vi "SMO.Dictionary.GetValue.vi"(6 "timeout (10ms)":i32=10, 8 "error in (no error)":errorcluster, 10 "Key":string, 11 "SMO.Dictionary":refnum<class "SMO.Dictionary.lvclass">) -> (0 "error out":errorcluster, 1 "Value":variant, 2 "Key":string, 3 "SMO.Dictionary out":refnum<class "SMO.Dictionary.lvclass">, 4 "timed out?":bool)   [LabVIEW 2013, in "SMO.Dictionary.lvlib" / "SMO.Dictionary.lvclass"]
doc: "---------------------------------------------------------------\nJKI State Machine Objects™\nhttp://jki.net/state-machine-objects/\nCopyright (C) 2005-2015, JKI <info@jki.net>\nALL RIGHTS RESERVEDJKI State Machine Objects (SMO) 1.0.0.4\nJKI - JKI\nCopyright (c) 2015, JKI"
uses:
  SMO.Dictionary.lvclass
  Typedefs/PrivateEvents--SMO.Dictionary.Get.ctl
  Typedefs/PrivateEvents--SMO.Dictionary.KeyValue-Pair.ctl
  <vilib>/JKI/JKI SMO/SMO/SMO.lvclass
panel:
  # "For instructions on how to use the JKI State Machine Objects, examples and video tutorials, visit:\nhttp://jki.net/state-machine-objects/\n\nJKI State Machine Objects™\nhttp://jki.net/state-machine-objects/\nCopyright (C) 2005-2015, JKI <info@jki.net>\nALL RIGHTS RESERVED"
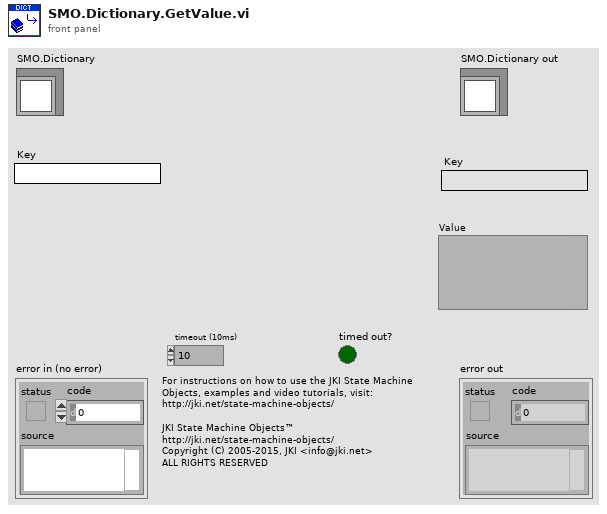
[diagram p1: front panel]
types:
  T1 = typedef "SMO.lvclass/SMOState --Enum.ctl" = enum16{"unknown", "Created", "Started", "Stopped"}
  T2 = typedef "SMO.Dictionary.lvlib/SMO.Dictionary.lvclass/PrivateEvents--SMO.Dictionary.KeyValue-Pair.ctl" = cluster{"Key":string, "Value":variant}
  T3 = typedef "SMO.Dictionary.lvlib/SMO.Dictionary.lvclass/PrivateEvents--SMO.Dictionary.Get.ctl" = cluster{"Key":string, "response":refnum<notifier>}
  T4 = typedef "SMO.Dictionary.lvlib/SMO.Dictionary.lvclass/PrivateEvents--Cluster.ctl" = cluster{"Update":refnum<user-event>, "Clear Dictionary":refnum<user-event>, "Delete":refnum<user-event>, "Get":refnum<user-event>, "GetMultiple":refnum<user-event>}
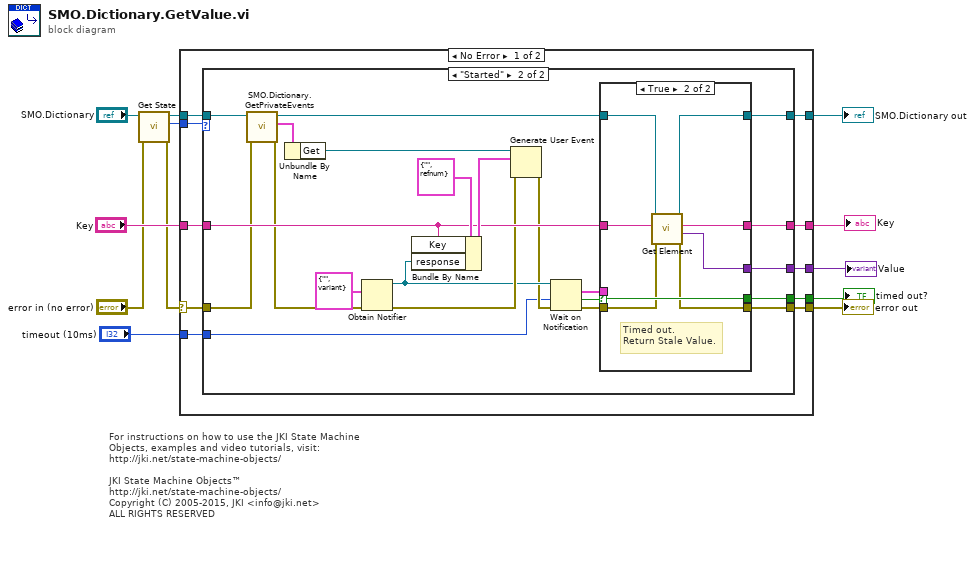
[diagram p0: block diagram]
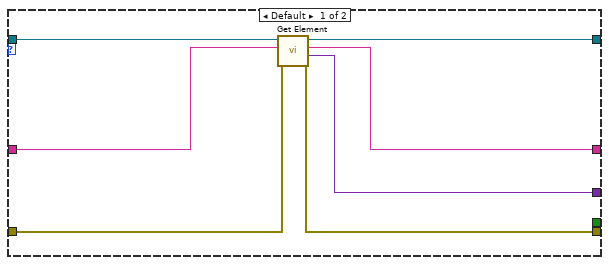
[diagram p2: hidden frame]
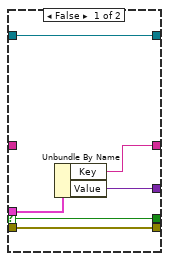
[diagram p3: hidden frame]
diagram:
  # "For instructions on how to use the JKI State Machine Objects, examples and video tutorials, visit:\nhttp://jki.net/state-machine-objects/\n\nJKI State Machine Objects™\nhttp://jki.net/state-machine-objects/\nCopyright (C) 2005-2015, JKI <info@jki.net>\nALL RIGHTS RESERVED"
  n1 = call <vilib>:"Get State.vi"("error in (no error)"="error in (no error)", "SMO"="SMO.Dictionary") -> ("error out"=w1:errorcluster, "SMO State"=w2:T1, "SMO out"=w3:refnum<class "SMO.Dictionary.lvclass">)  [unwired: 7 in]
  n2 = case shown="No Error" w1 {
    selector: w1 -> [w13 w67]
    tunnel: [w22 w68] -> w12
    tunnel: [w21 w66] -> w11
    tunnel: [w20 _] -> w10
    tunnel: [w19 _] -> w9
    tunnel: [w18 w67] -> w8
    tunnel: "Key" -> [w17 w66]
    tunnel: "timeout (10ms)" -> [w16 _]
    tunnel: w3 -> [w15 w68]
    tunnel: w2 -> [w14 _]
    frame No Error {
      n3 = case shown="\"Started\"" w14 {
        tunnel: [w28 w46] -> w22
        tunnel: [w23 w45] -> w21
        tunnel: [w24 w44] -> w20
        tunnel: [_ w43] -> w19
        tunnel: [w25 w42] -> w18
        tunnel: w17 -> [w27 w41]
        tunnel: w16 -> [_ w35]
        tunnel: w13 -> [w26 w31]
        tunnel: w15 -> [w29 w30]
        frame Default {
          n4 = call-dynamic "Get Element.vi"("error in (no error)"=w26, "Key"=w27, "SMO.Dictionary in"=w29) -> ("error out"=w25:errorcluster, "Value"=w24:variant, "Key dup"=w23:string, "SMO.Dictionary out"=w28:refnum<class "SMO.Dictionary.lvclass">)  [unwired: 5 in]
        }
        frame "Started" {
          n5 = call "SMO.Dictionary.GetPrivateEvents.vi"("error in (no error)"=w31, "SMO.Dictionary"=w30) -> ("error out"=w39:errorcluster, "Private Events"=w51:T4, "SMO.Dictionary out"=w47:refnum<class "SMO.Dictionary.lvclass">)  [unwired: 7 in]
          n6 = Unbundle By Name(w51) -> ("Get"=w48:refnum<user-event>)
          n7 = Obtain Notifier(notification data type=T2 {"Key"="", "Value"=variant} ("Update"), error in (no error)=w39) -> (notifier out=w37:refnum<notifier>, error out=w38:errorcluster)  [unwired: 2 in, 1 out]
          n8 = Bundle By Name(cluster=T3 {"Key"="", "response"=refnum} ("Get"), "Key"=w41, "response"=w37) -> (w49:T3)
          n9 = Generate User Event(user event=w48, event data cluster=w49, error in=w38) -> (error out=w36:errorcluster)  [unwired: 1 in, 1 out]
          n10 = Wait on Notification(notifier=w37, timeout in ms (-1)=w35, error in (no error)=w36) -> (notification=w32:T2, timed out?=w33:bool, error out=w34:errorcluster)  [unwired: 1 in, 1 out]
          n11 = case shown="True" w33 {
            selector: w33 -> [w55 w65]
            tunnel: w47 -> [w57 w64]
            tunnel: [w57 w63] -> w46
            tunnel: w34 -> [w56 w59]
            tunnel: [w56 w60] -> w42
            tunnel: [w55 w65] -> w43
            tunnel: [w54 w62] -> w45
            tunnel: [w53 w61] -> w44
            tunnel: w32 -> [w52 _]
            tunnel: w41 -> [_ w58]
            frame False {
              n12 = Unbundle By Name(w52) -> ("Key"=w54:string, "Value"=w53:variant)
            }
            frame True {
              # "Timed out.\nReturn Stale Value."
              n13 = call-dynamic "Get Element.vi"("error in (no error)"=w59, "Key"=w58, "SMO.Dictionary in"=w64) -> ("error out"=w60:errorcluster, "Value"=w61:variant, "Key dup"=w62:string, "SMO.Dictionary out"=w63:refnum<class "SMO.Dictionary.lvclass">)  [unwired: 5 in]
            }
          }
        }
      }
    }
    frame Error {
    }
  }
  "error out" <- w8
  "SMO.Dictionary out" <- w12
  "Value" <- w10
  "Key" <- w11
  "timed out?" <- w9
